vi "ELMOS Set Speed.vi"(9 "SpeedHz":u32, 10 "LINChannel":u8, 11 "DeviceHandle":i32) -> (3 "function return":i32)   [LabVIEW 2010, in "elmos_programer.lvlib"]
doc: "int WINAPI ELMOS_SetSpeed(int DeviceHandle, unsigned char LINChannel, unsigned int SpeedHz);"
uses:
  elmos_programer.lvlib
  USB2XXX/trunk/USB2XXX/USB2XXX/vs2019/Release/USB2XXX.dll
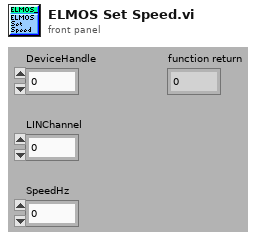
[diagram p1: front panel]
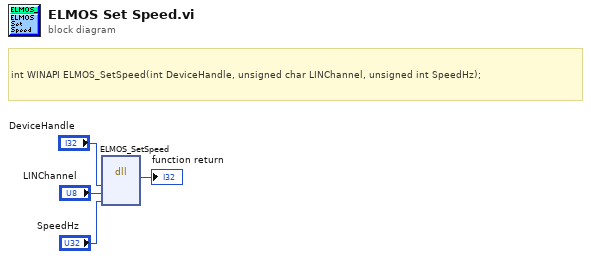
[diagram p0: block diagram]
diagram:
  # "int WINAPI ELMOS_SetSpeed(int DeviceHandle, unsigned char LINChannel, unsigned int SpeedHz);"
  n1 = dll-call lib="E:/Projects/USB2XXX/trunk/USB2XXX/USB2XXX/vs2019/Release/USB2XXX.*" fn="ELMOS_SetSpeed"("DeviceHandle"="DeviceHandle", "LINChannel"="LINChannel", "SpeedHz"="SpeedHz") -> (→"function return":i32)  [unwired: 6 in, 2 out]
